vi "main1.vi"() -> ()   [LabVIEW 2022 SP3]
uses:
  Control 1.ctl
  <vilib>/numeric/Random Number (Range) DBL.vi
panel:
  out "Wrota zamkniete":bool
  in  "Stopien zamkniecia wrot 2":dbl(slide) scale=0.0..10.0
  in  "Poziom zamkniecia wrot 1":dbl(slide) scale=0.0..10.0
  in  "Start sluza proces":bool
  in  "stop":bool
  out "Poziom wody za sluza":dbl(slide)=8.064516129032258 scale=0.0..10.0
  out "Poziom wody w sluzie":dbl(slide)=4.0 scale=0.0..10.0
  out "Poziom wody przed sluza":dbl(slide)=4.129032258064516 scale=0.0..10.0
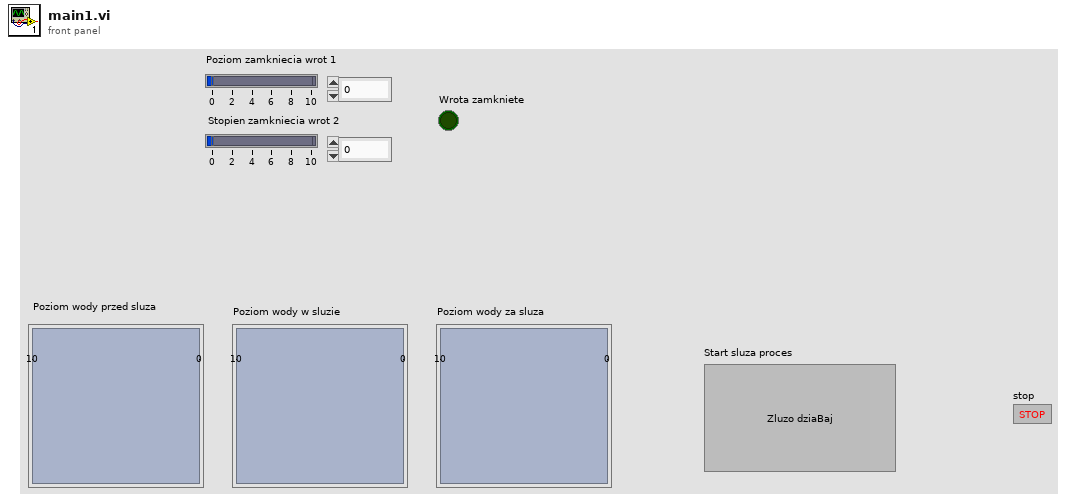
[diagram p1: front panel]
types:
  T1 = enum8{"Enabled", "Disabled", "Disabled and Grayed Out"}
  T2 = typedef "Control 1.ctl" = enum16{"Init", "Idle", "Monitor", "Process", "Exit"}
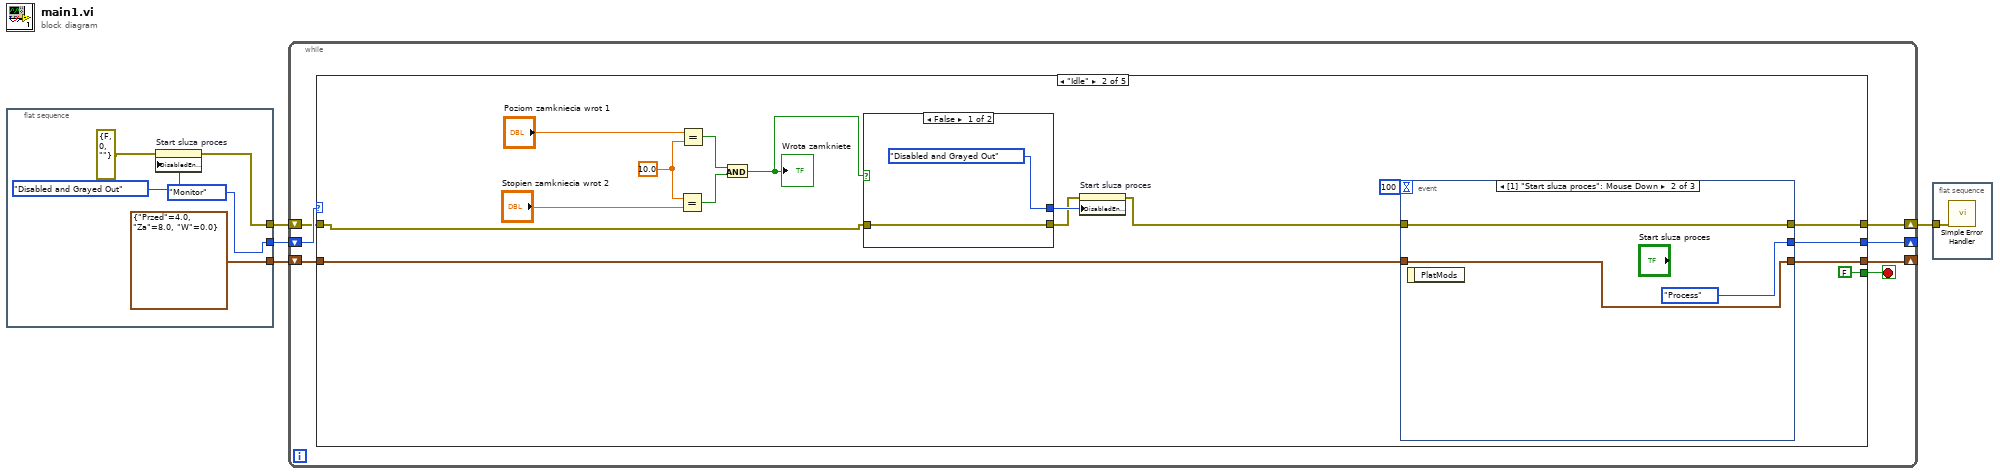
[diagram p0: block diagram]
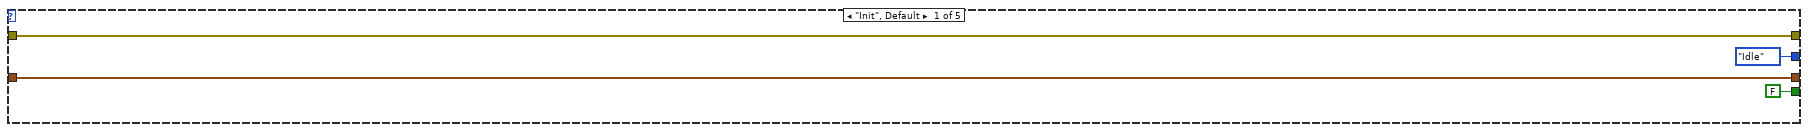
[diagram p2: hidden frame]
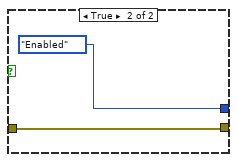
[diagram p3: hidden frame]
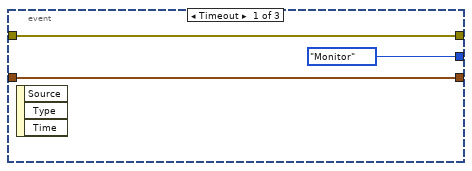
[diagram p4: hidden frame]
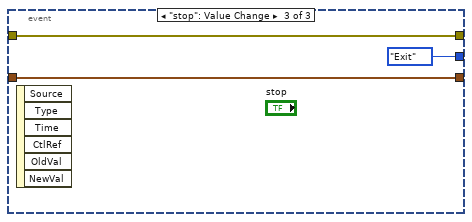
[diagram p5: hidden frame]
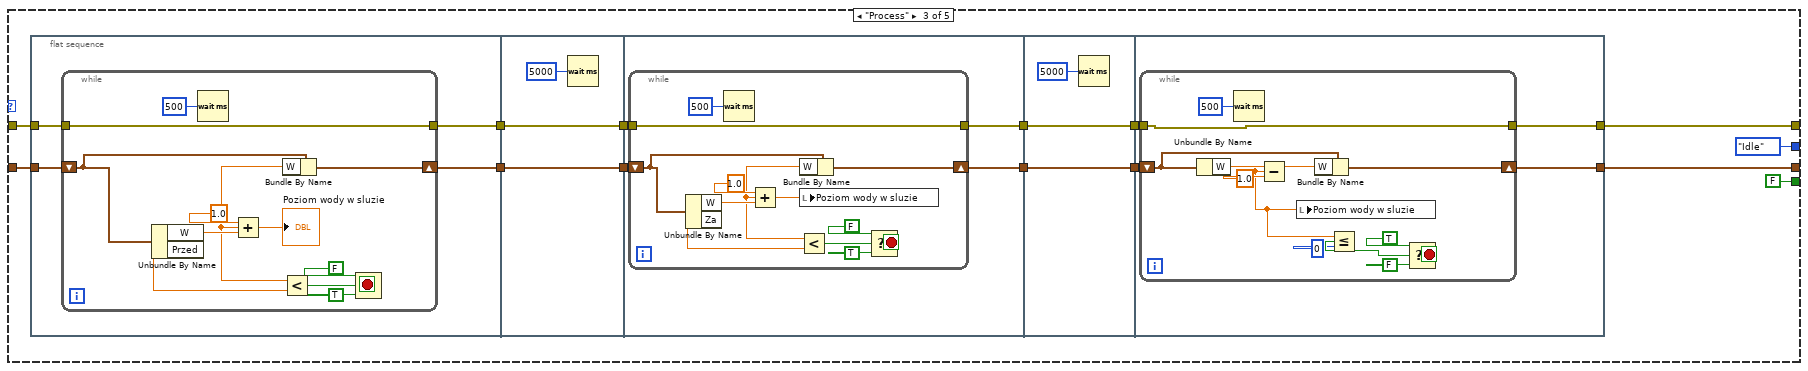
[diagram p6: hidden frame]
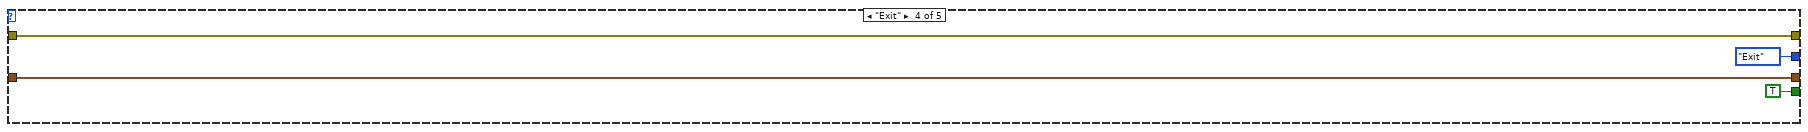
[diagram p7: hidden frame]
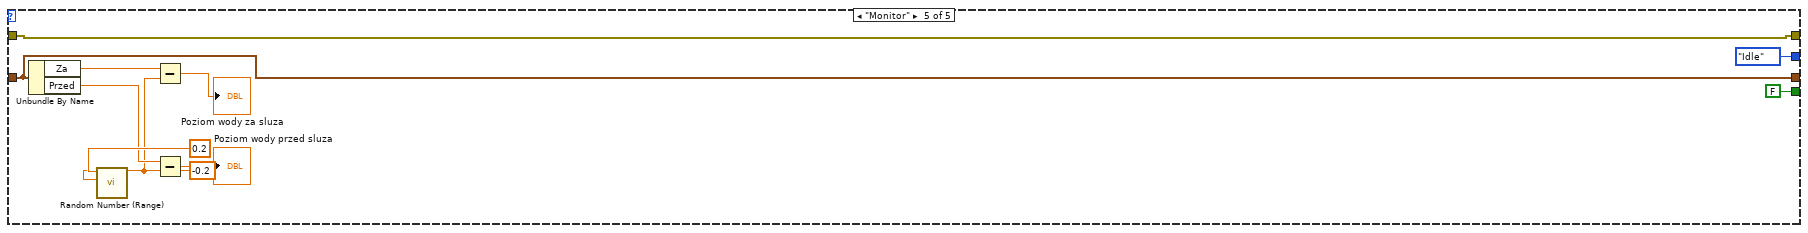
[diagram p8: hidden frame]
diagram:
  n1 = flat-sequence {
    tunnel: [cluster{"Przed":dbl, "Za":dbl, "W":dbl} {"Przed"=4.0, "Za"=8.0, "W"=0.0}] -> w4
    tunnel: [Control_1."Monitor"] -> w3
    tunnel: [w6] -> w2
    frame #0 {
      n2 = property on="Start sluza proces" class="Bool (strict)"(error in=errorcluster {"status"=FALSE, "code"=0, "source"=""} ("error constant"), "DisabledEnum"=T1."Disabled and Grayed Out" ("Disabled")) -> (error out=w6:errorcluster)  [unwired: 1 in, 1 out]
    }
  }
  n3 = while {
    shift-right: [w11] -> w1
    shift-left: w2 -> [w10]
    shift-right: [w15] -> _
    shift-left: w4 -> [w14]
    shift-right: [w13] -> _
    shift-left: w3 -> [w16]
    stop <- w12 stop-if-true
    n4 = case shown="\"Idle\"" w16 {
      tunnel: [w20 w33 w54 w119 w125] -> w15
      tunnel: w14 -> [w20 w32 w61 w119 w125]
      tunnel: [Control_1."Idle" w34 Control_1."Idle" Control_1."Exit" Control_1."Idle"] -> w13
      tunnel: [FALSE FALSE FALSE TRUE FALSE] -> w12
      tunnel: [w17 w31 w58 w118 w126] -> w11
      tunnel: w10 -> [w17 w25 w60 w118 w126]
      frame "Init", Default {
      }
      frame "Idle" {
        w26 = 10.0
        n5 = Equal?(x=w26, y="Stopien zamkniecia wrot 2") -> (x = y?=w28:bool)
        n6 = Equal?(x="Poziom zamkniecia wrot 1", y=w26) -> (x = y?=w29:bool)
        n7 = And(x=w29, y=w28) -> (x .and. y?=w24:bool)
        "Wrota zamkniete" <- w24
        n8 = case shown="False" w24 {
          tunnel: w25 -> [w38 w39]
          tunnel: [w38 w39] -> w21
          tunnel: [T1."Disabled and Grayed Out" ("Disabled") T1."Enabled" ("Disabled")] -> w23
          frame False {
          }
          frame True {
          }
        }
        n9 = property on="Start sluza proces" class="Bool (strict)"(error in=w21, "DisabledEnum"=w23) -> (error out=w22:errorcluster)  [unwired: 1 in, 1 out]
        n10 = event shown="[1] \"Start sluza proces\": Mouse Down" {
          selector: _ -> [_ _ _]
          dyn-events: _ -> [_ _ _]
          timeout: 100 -> [_ _ _]
          tunnel: [Control_1."Monitor" Control_1."Process" Control_1."Exit"] -> w34
          tunnel: [w42 w45 w49] -> w33
          tunnel: w32 -> [w42 w45 w49]
          tunnel: [w41 w44 w47] -> w31
          tunnel: w22 -> [w41 w44 w47]
          event Timeout {
            n11 = event-data() -> ()  [unwired: 1 in, 3 out]
          }
          event "Start sluza proces": Mouse Down {
            n12 = event-data() -> ()  [unwired: 1 in, 1 out]
          }
          event "stop": Value Change {
            n13 = event-data() -> ()  [unwired: 1 in, 6 out]
          }
        }
      }
      frame "Process" {
        n14 = flat-sequence {
          tunnel: w61 -> [w67]
          tunnel: w60 -> [w66]
          tunnel: [w65] -> w59
          tunnel: [w64] -> w57
          tunnel: w59 -> [w81]
          tunnel: w57 -> [w80]
          tunnel: [w81] -> w56
          tunnel: [w80] -> w55
          tunnel: w56 -> [w84]
          tunnel: w55 -> [w86]
          tunnel: [w85] -> w53
          tunnel: [w83] -> w52
          tunnel: w53 -> [w101]
          tunnel: w52 -> [w100]
          tunnel: [w101] -> w51
          tunnel: [w100] -> w50
          tunnel: [w104] -> w54
          tunnel: [w102] -> w58
          tunnel: w51 -> [w103]
          tunnel: w50 -> [w105]
          frame #0 {
            n15 = while {
              shift-right: [w74] -> w65
              shift-left: w67 -> [w75]
              tunnel: [w77] -> w64
              tunnel: w66 -> [w77]
              stop <- w69 stop-if-true
              n16 = Unbundle By Name(w75) -> ("W"=w78:dbl, "Przed"=w73:dbl)
              n17 = Wait (ms)(milliseconds to wait=u32 500) -> ()  [unwired: 1 out]
              n18 = Add(x=1.0, y=w78) -> (x+y=w68:dbl)
              "Poziom wody w sluzie" <- w68
              n19 = Less?(x=w68, y=w73) -> (x < y?=w72:bool)
              n20 = Bundle By Name(cluster=w75, "W"=w68) -> (w74:cluster{"Przed":dbl, "Za":dbl, "W":dbl})
              n21 = Select(t=FALSE, s=w72, f=TRUE) -> (s? t:f=w69:bool)
            }
          }
          frame #1 {
            n22 = Wait (ms)(milliseconds to wait=u32 5000) -> ()  [unwired: 1 out]
          }
          frame #2 {
            n23 = while {
              tunnel: [w98] -> w85
              tunnel: w86 -> [w98]
              shift-right: [w94] -> w83
              shift-left: w84 -> [w93]
              stop <- w89 stop-if-true
              n24 = Unbundle By Name(w93) -> ("W"=w92:dbl, "Za"=w90:dbl)
              n25 = Wait (ms)(milliseconds to wait=u32 500) -> ()  [unwired: 1 out]
              n26 = Add(x=1.0, y=w92) -> (x+y=w88:dbl)
              n27 = Less?(x=w88, y=w90) -> (x < y?=w97:bool)
              n28 = Bundle By Name(cluster=w93, "W"=w88) -> (w94:cluster{"Przed":dbl, "Za":dbl, "W":dbl})
              n29 = local write "Poziom wody w sluzie"(w88) -> ()
              n30 = Select(t=FALSE, s=w97, f=TRUE) -> (s? t:f=w89:bool)
            }
          }
          frame #3 {
            n31 = Wait (ms)(milliseconds to wait=u32 5000) -> ()  [unwired: 1 out]
          }
          frame #4 {
            n32 = while {
              tunnel: w103 -> [w117]
              tunnel: [w117] -> w102
              shift-right: [w107] -> w104
              shift-left: w105 -> [w109]
              stop <- w110 stop-if-true
              n33 = Unbundle By Name(w109) -> ("W"=w116:dbl)
              n34 = Wait (ms)(milliseconds to wait=u32 500) -> ()  [unwired: 1 out]
              n35 = Subtract(x=w116, y=1.0) -> (x-y=w108:dbl)
              n36 = local write "Poziom wody w sluzie"(w108) -> ()
              n37 = Bundle By Name(cluster=w109, "W"=w108) -> (w107:cluster{"Przed":dbl, "Za":dbl, "W":dbl})
              n38 = Less Or Equal?(x=w108, y=0) -> (x <= y?=w114:bool)
              n39 = Select(t=TRUE, s=w114, f=FALSE) -> (s? t:f=w110:bool)
            }
          }
        }
      }
      frame "Exit" {
      }
      frame "Monitor" {
        n40 = Unbundle By Name(w125) -> ("Za"=w128:dbl, "Przed"=w129:dbl)
        n41 = call-poly <vilib>:"Random Number (Range).vi"("lower bound (0)"=-0.2, "upper bound (100)"=0.2) -> ("number"=w127:dbl)  [unwired: 9 in]
        n42 = Subtract(x=w128, y=w127) -> (x-y=→"Poziom wody za sluza":dbl)
        n43 = Subtract(x=w129, y=w127) -> (x-y=→"Poziom wody przed sluza":dbl)
      }
    }
  }
  n44 = flat-sequence {
    tunnel: w1 -> [w133]
    frame #0 {
      n45 = call <vilib>:"Simple Error Handler.vi"("error in (no error)"=w133) -> ()  [unwired: 4 in, 5 out]
    }
  }
